vi "StateScalarStateColorStateName.vi"() -> ()   [LabVIEW 2014, in "examples.lvlib"]
uses:
  vis/tango_vi.llb/_TangoReadStateScalarAttribute.vi
  examples.lvlib
  vis/tango_vi.llb/tango.lvlib
panel:
  in  "<TangoTest> device name":string="sys/tg_test/1"
  out "State Name":string
  out "State Color":u32(colorbox)=16448250
  out "State Code":u32
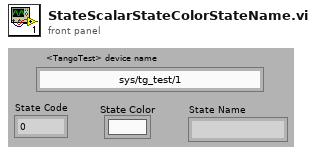
[diagram p1: front panel]
types:
  T1 = typedef "tango.lvlib/_TangoState_t.ctl" = enum32{"ON", "OFF", "CLOSE", "OPEN", "INSERT", "EXTRACT", "MOVING", "STANDBY", "FAULT", "INIT", "RUNNING", "ALARM", "DISABLE", "UNKNOWN"}
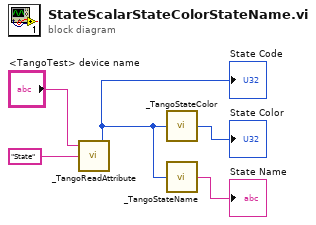
[diagram p0: block diagram]
diagram:
  n1 = call-poly "_TangoReadAttribute.vi"("attribute name"="State", "device name"="<TangoTest> device name") -> ("value"=w2:T1)  [unwired: 1 in, 2 out]
  "State Code" <- w2
  n2 = call "_TangoStateColor.vi"("State"=w2) -> ("State Color"=→"State Color":u32)
  n3 = call "_TangoStateName.vi"("State"=w2) -> ("State Name"=→"State Name":string)
